vi "Active Plugins.vi"(8 "error in (no error)":errorcluster, 11 "Framework in":refnum<class "Framework.lvclass">) -> (0 "error out":errorcluster, 3 "Framework out":refnum<class "Framework.lvclass">)   [LabVIEW 2017, in "DSF Core.lvlib" / "Framework.lvclass"]
uses:
  Framework.lvclass
  Framework.lvclass/Framework.ctl
  Plugin/Plugin.lvclass/Plugin.ctl
  Timing/Timing.lvclass/Timing.ctl
  State/Framework State.lvclass/Framework State.ctl
  Plugin/Get Timing.vi
  Timing/Is Active Cycle.vi
  Timing/Get Decimation.vi
  Timing/Get Offset.vi
  Plugin/Plugin.lvclass
  State/Framework State.lvclass
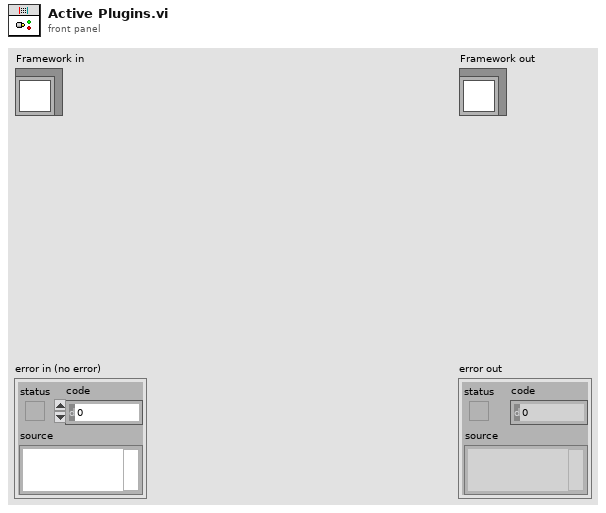
[diagram p1: front panel]
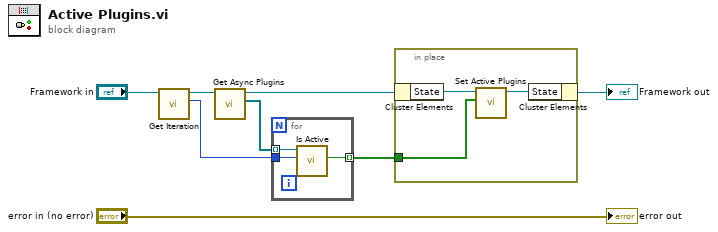
[diagram p0: block diagram]
diagram:
  n1 = call "Get Iteration.vi"("Framework in"="Framework in") -> ("iteration"=w4:u64, "Framework out"=w6:refnum<class "Framework.lvclass">)  [unwired: 9 in]
  n2 = call "Get Async Plugins.vi"("Framework in"=w6) -> ("Plugins"=w5:refnum<class "Plugin.lvclass">[], "Framework out"=w3:refnum<class "Framework.lvclass">)  [unwired: 9 in]
  n3 = for {
    tunnel: w5 -> [w11] mode=indexing
    tunnel: [w10] -> w2 mode=indexing
    tunnel: w4 -> [w9]
    n4 = call "Is Active.vi"("cycle count"=w9, "Plugin in"=w11) -> ("active this cycle?"=w10:bool)  [unwired: 8 in, 1 out]
  }
  n5 = in-place {
    in-place-border: w2 -> [w12]
    n6 = in-place-cluster #1(w3) -> ("State"=w14:refnum<class "Framework State.lvclass">)
    n7 = call "Set Active Plugins.vi"("Active Plugins"=w12, "Framework State in"=w14) -> ("Framework State out"=w13:refnum<class "Framework State.lvclass">)  [unwired: 9 in]
    n8 = in-place-cluster #1("State"=w13) -> (→"Framework out":refnum<class "Framework.lvclass">)
  }
  "error out" <- "error in (no error)"
